vi "TracePoint_BadImage.vi"(8 "error in (no error)":errorcluster, 9 "histogram":u32[](array[numeric]), 10 "Camera":string, 11 "Qbus":refnum<class "Qbus.lvclass">) -> (0 "error out":errorcluster)   [LabVIEW 2017, in "IrAcquisition.lvlib"]
uses:
  <vilib>/addons/InsightCM/Devices/Shared/Ir/IrAcquisition/IrAcquisition.lvlib
  <vilib>/addons/Qbus/Qbus.lvclass
  <vilib>/addons/TraceLogger/TraceLogger.lvlib
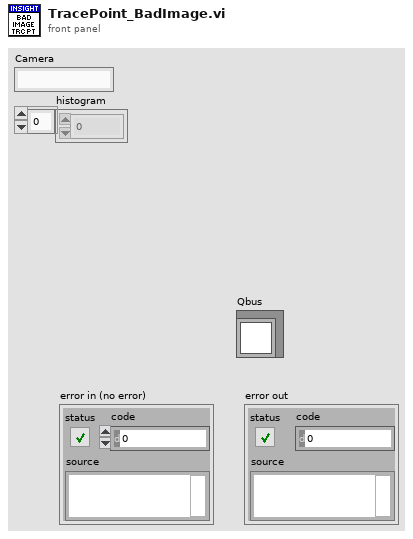
[diagram p1: front panel]
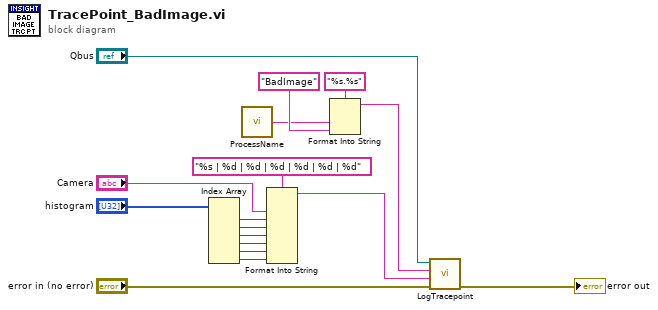
[diagram p0: block diagram]
diagram:
  n1 = Index Array(array="histogram") -> (element #1=w5:u32, element #2=w6:u32, element #3=w7:u32, element #4=w8:u32, element #5=w9:u32, element #6=w10:u32)  [unwired: 6 in]
  n2 = call <vilib>:"ProcessName.vi"() -> ("process name"=w11:string)  [unwired: 5 in]
  n3 = Format Into String(format string="%s | %d | %d | %d | %d | %d | %d", "Camera", w5, w6, w7, w8, w9, w10) -> (resulting string=w2:string)  [unwired: 2 in, 1 out]
  n4 = Format Into String(format string="%s.%s", w11, "BadImage" ("tracepoint")) -> (resulting string=w12:string)  [unwired: 2 in, 1 out]
  n5 = call <vilib>:"LogTracepoint.vi"("error in (no error)"="error in (no error)", "log string"=w2, "tracepoint"=w12, "qbus in"="Qbus") -> ("error out"=→"error out":errorcluster)  [unwired: 6 in, 1 out]
